vi "FTW-EventLogger-CreateObserver.vi"(0 "Event Logger API":refnum<class "FTW-EventLogger-API.lvclass">, 11 "error in":errorcluster) -> (4 "Event Logger API out":refnum<class "FTW-EventLogger-API.lvclass">, 6 "Logged Event Registration":refnum<event-registration>, 15 "error out":errorcluster)   [LabVIEW 2014, in "FTW-EventLogger-API.lvclass"]
doc: "This method create a new Event Registration for the given Logger Process specified by LoggerID.\n\nWhen new log events are added to the Logger, they will also be relayed to this Observer. Note that an Observer will very likely receive this relayed Log Event before it's actually logged by the Logger.\n\nAny number of Observers may be created. Each Observer must be explicitly closed by your application; destroying the Logger does not destroy a Log Observer. It's recommended that a Log Observer is wired to an Event Handler Structure, since unhandled events continue to enqueue indefinitely if not handled."
uses:
  FTW-EventLogger-API.lvclass
panel:
  # "Inputs"
  # "Outputs"
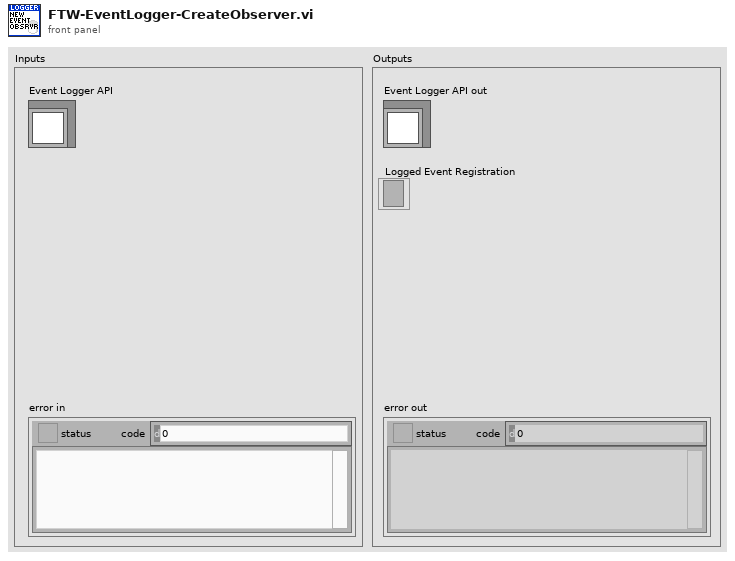
[diagram p1: front panel]
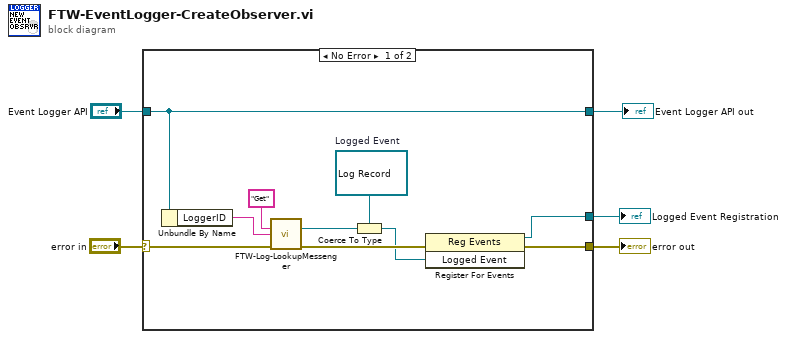
[diagram p0: block diagram]
diagram:
  n1 = case shown="No Error" "error in" {
    selector: "error in" -> [w15 w17]
    tunnel: [w13 w17] -> w5
    tunnel: [w10 _] -> w3
    tunnel: [w7 w16] -> w2
    tunnel: "Event Logger API" -> [w7 w16]
    frame No Error {
      w11 = refnum<user-event> refnum  # Logged Event
      n2 = Unbundle By Name(w7) -> ("LoggerID"=w6:string)
      n3 = call "FTW-Log-LookupMessenger.vi"("Action"="Get", "LoggerID"=w6, "error in"=w15) -> ("Logged Event Broadcast"=w9:refnum<user-event>, "error out"=w14:errorcluster)  [unwired: 9 in, 2 out]
      n4 = Coerce To Type(0:w9, 1:w11) -> (2:w12:refnum<user-event>)
      n5 = register-events(error in=w14, w12) -> (reference out=w10:refnum<event-registration>, error out=w13:errorcluster)  [unwired: 1 in]
    }
    frame Error {
    }
  }
  "error out" <- w5
  "Logged Event Registration" <- w3
  "Event Logger API out" <- w2
